vi "Longi.vi"(8 "error in (no error)":errorcluster) -> (0 "error out":errorcluster, 3 "function return":dbl)   [LabVIEW 2014, in "MASTTCSGET.lvlib"]
doc: "this is longtitude of udaipur\n\n\n\n__declspec (dllexport) float Longi();"
uses:
  MASTTCSGET.lvlib
  MASTTCSGET.dll
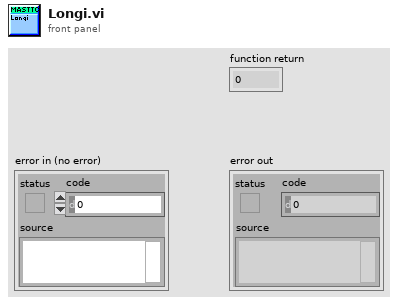
[diagram p1: front panel]
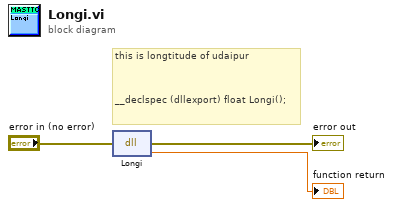
[diagram p0: block diagram]
diagram:
  # "this is longtitude of udaipur\n\n\n\n__declspec (dllexport) float Longi();"
  n1 = dll-call lib="C:/Users/sanjay/Desktop/mast_controlsystem/MASTTCSGET.*" fn="Longi"(error in="error in (no error)") -> (error out=→"error out":errorcluster, →"function return":dbl)  [unwired: 2 in, 1 out]
